vi "Write Full Layer.vi"(8 "Error In":errorcluster, 11 "Database Full Information In":T1 {"Database Write Information"."Layer Information Array"."Deposition Method" items=["Blade Coating", "Spin Coating", "Thermal Evaporation", "E-Beam Evaporation", "Sputtering", "Drop Casting", "Dip Coating", "Pulsed Laser Deposition", "Chemival Vapour Deposition", "Atomic Layer Deposition", "Spray Coating", "Screen Printing", "Electroplating", "Molecular Beam Epitaxy", "Custom Deposition"]; "Database Write Information"."Layer Information Array"."Layer Type" items=["Front Electrode", "Electron Transport Layer", "Active Layer", "Hole Transport Layer", "Back Electrode", "Custom Layer"]}) -> (0 "Error Out":errorcluster, 3 "Database Full Information Out":T1 {"Database Write Information"."Layer Information Array"."Deposition Method" items=["Blade Coating", "Spin Coating", "Thermal Evaporation", "E-Beam Evaporation", "Sputtering", "Drop Casting", "Dip Coating", "Pulsed Laser Deposition", "Chemival Vapour Deposition", "Atomic Layer Deposition", "Spray Coating", "Screen Printing", "Electroplating", "Molecular Beam Epitaxy", "Custom Deposition"]; "Database Write Information"."Layer Information Array"."Layer Type" items=["Front Electrode", "Electron Transport Layer", "Active Layer", "Hole Transport Layer", "Back Electrode", "Custom Layer"]})   [LabVIEW 2020]
uses:
  Data Clusters/Database Information.ctl
  Data Clusters/Layer Information Cluster.ctl
  <vilib>/addons/database/Connection.llb/Conn ObjectReference.ctl
  <vilib>/addons/database/NI_Database_API.lvlib
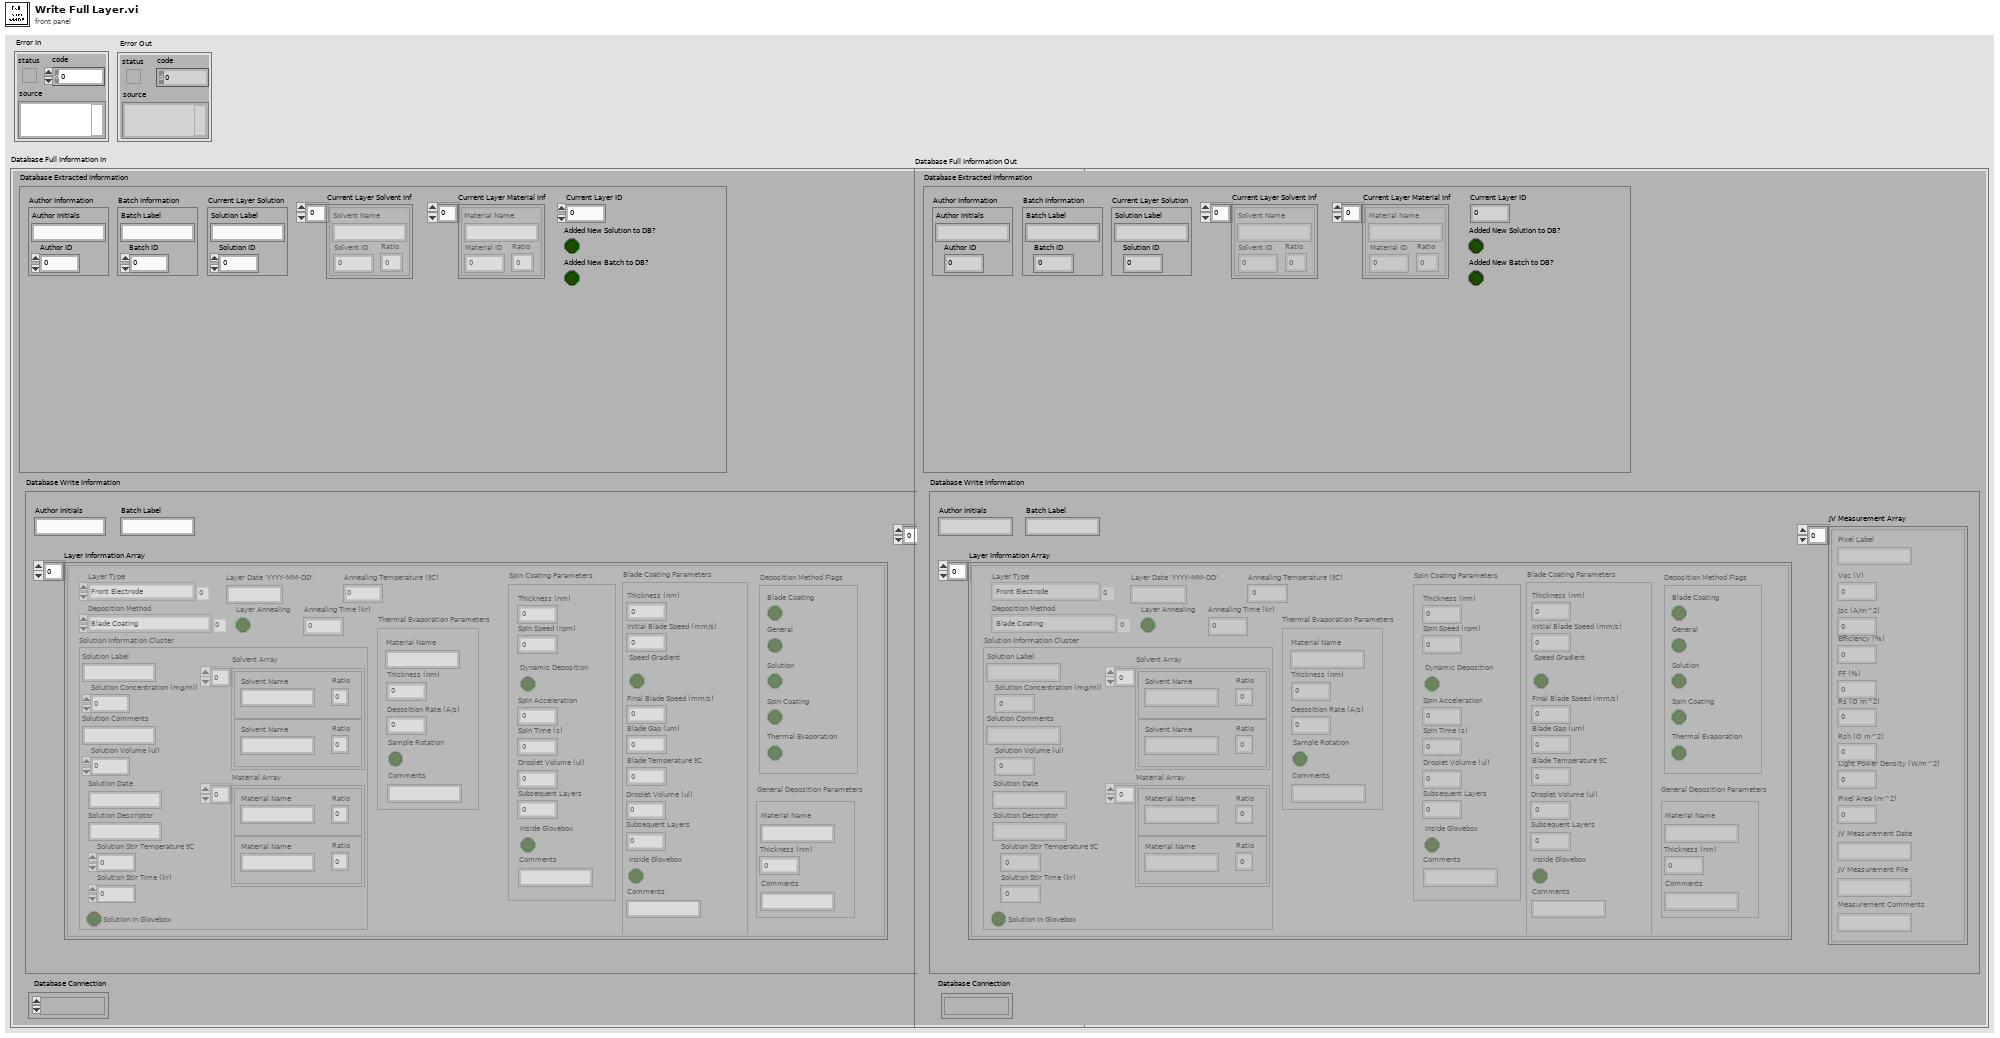
[diagram p1: front panel]
types:
  T1 = typedef "Database Information.ctl" = cluster{"Database Extracted Information":cluster{"Author Information":cluster{"Author Initials":string, "Author ID":i32}, "Batch Information":cluster{"Batch Label":string, "Batch ID":i32}, "Current Layer Solution":cluster{"Solution Label":string, "Solution ID":i32}, "Current Layer ID":i32, "Current Layer Solvent Inf":cluster{"Solvent Name":string, "Solvent ID":i32, "Ratio":dbl}[], "Current Layer Material Inf":cluster{"Material Name":string, "Material ID":i32, "Ratio":dbl}[], "Added New Solution to DB?":bool, "Added New Batch to DB?":bool}, "Database Write Information":cluster{"Author Initials":string, "Batch Label":string, "Layer Information Array":T2[], "JV Measurement Array":cluster{"Pixel Label":string, "Voc (V) ":dbl, "Jsc (A/m^2) ":dbl, "Efficiency (%)":dbl, "FF (%)":dbl, "Rs (O m^2)":dbl, "Rsh (O m^2)":dbl, "Light Power Density (W/m^2)":dbl, "Pixel Area (m^2)":dbl, "JV Measurement Date":string, "JV Measurement File":string, "Measurement Comments":string}[]}, "Database Connection":T3}
  T2 = typedef "Layer Information Cluster.ctl" = cluster{"Solution Information Cluster":cluster{"Solution Label":string, "Solution Concentration (mg/ml)":dbl, "Solution Comments ":string, "Solution Volume (ul) ":dbl, "Solution Date ":string, "Solution Descriptor ":string, "Solution Stir Temperature ºC ":dbl, "Solution Stir Time (kr) ":dbl, "Solution In Glovebox":bool, "Solvent Array":cluster{"Solvent Name":string, "Ratio":dbl}[], "Material Array":cluster{"Material Name":string, "Ratio":dbl}[]}, "Layer Type":u16, "Deposition Method":u16, "Layer Annealing":bool, "General Deposition Parameters":cluster{"Thickness (nm)":dbl, "Comments":string, "Material Name":string}, "Blade Coating Parameters":cluster{"Thickness (nm)":dbl, "Initial Blade Speed (mm/s)":dbl, "Speed Gradient":bool, "Final Blade Speed (mm/s)":dbl, "Blade Gap (um)":dbl, "Droplet Volume (ul)":dbl, "Subsequent Layers":dbl, "Inside Glovebox":bool, "Comments":string, "Blade Temperature ºC":dbl}, "Spin Coating Parameters":cluster{"Thickness (nm)":dbl, "Spin Speed (rpm)":dbl, "Dynamic Deposition":bool, "Spin Acceleration":dbl, "Spin Time (s)":dbl, "Droplet Volume (ul)":dbl, "Subsequent Layers":dbl, "Inside Glovebox":bool, "Comments":string}, "Thermal Evaporation Parameters":cluster{"Deposition Rate (A/s)":dbl, "Thickness (nm)":dbl, "Comments":string, "Material Name":string, "Sample Rotation":bool}, "Layer Date 'YYYY-MM-DD'":string, "Annealing Time (kr)":dbl, "Annealing Temperature (ºC)":dbl, "Deposition Method Flags":cluster{"Blade Coating":bool, "General ":bool, "Solution":bool, "Spin Coating":bool, "Thermal Evaporation":bool}}
  T3 = typedef "NI_Database_API.lvlib/Conn ObjectReference.ctl" = refnum<k1>
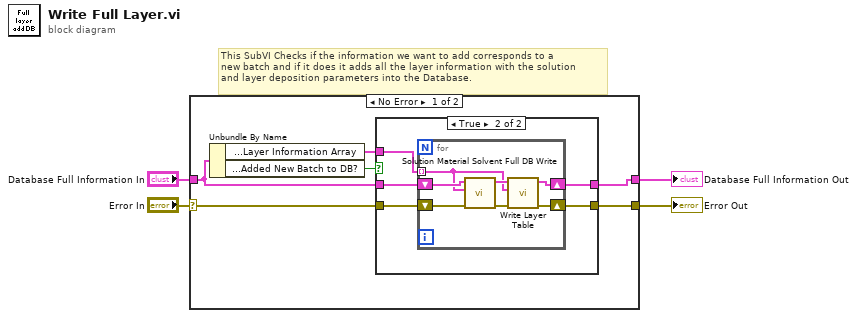
[diagram p0: block diagram]
diagram:
  # "This SubVI Checks if the information we want to add corresponds to a \nnew batch and if it does it adds all the layer information with the solution\nand layer deposition parameters into the Database."
  n1 = case shown="No Error" "Error In" {
    selector: "Error In" -> [w9 w26]
    tunnel: [w7 w26] -> w3
    tunnel: "Database Full Information In" -> [w8 w25]
    tunnel: [w6 w25] -> w1
    frame No Error {
      n2 = Unbundle By Name(w8) -> ("Database Write Information.Layer Information Array"=w10:T2[], "Database Extracted Information.Added New Batch to DB?"=w5:bool)
      n3 = case shown="True" w5 {
        tunnel: w10 -> [_ w17]
        tunnel: w9 -> [w11 w16]
        tunnel: w8 -> [w12 w15]
        tunnel: [w11 w14] -> w7
        tunnel: [w12 w13] -> w6
        frame False {
        }
        frame True {
          n4 = for {
            tunnel: w17 -> [w18] mode=indexing
            shift-right: [w21] -> w14
            shift-left: w16 -> [w24]
            shift-right: [w19] -> w13
            shift-left: w15 -> [w23]
            n5 = call "Solution Material Solvent Full DB Write.vi"("error in (no error)"=w24, "Layer Information Array"=w18, "Database Full Information In"=w23) -> ("error out"=w22:errorcluster, "Database Full Information Out"=w20:T1)  [unwired: 7 in]
            n6 = call "Write Layer Table.vi"("Error In"=w22, "Layer Information Cluster"=w18, "Database Full Information In"=w20) -> ("Error Out"=w21:errorcluster, "Database Full Information Out"=w19:T1)  [unwired: 7 in]
          }
        }
      }
    }
    frame Error {
    }
  }
  "Error Out" <- w3
  "Database Full Information Out" <- w1
